vi "BuildClass.vi"(6 "ProjectPath":path, 7 "Parent":enum16{"None", "Interface", "Class"}(ring)=enum."Interface", 8 "error in (no error)":errorcluster, 9 "Application":refnum<vi>, 10 "ParentRef":refnum<vi>, 11 "Class in":refnum<class "Class.lvclass">) -> (0 "error out":errorcluster, 3 "Class out":refnum<class "Class.lvclass">)   [LabVIEW 2020, in "Mermaid.lvlib" / "Class.lvclass"]
uses:
  Class.lvclass
  Class.lvclass/Class.ctl
  _CreateClass/CreateClass.lvclass
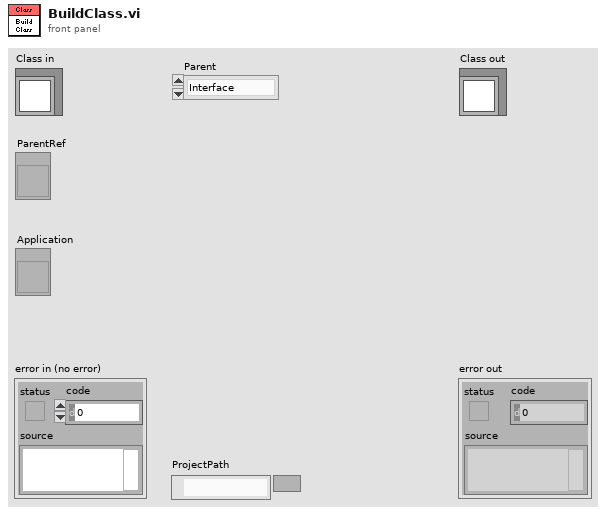
[diagram p1: front panel]
types:
  T1 = typedef "Mermaid.lvlib/ParseMermaid.lvclass/Attributes.ctl" = cluster{"Name":string, "Type":i32}[]
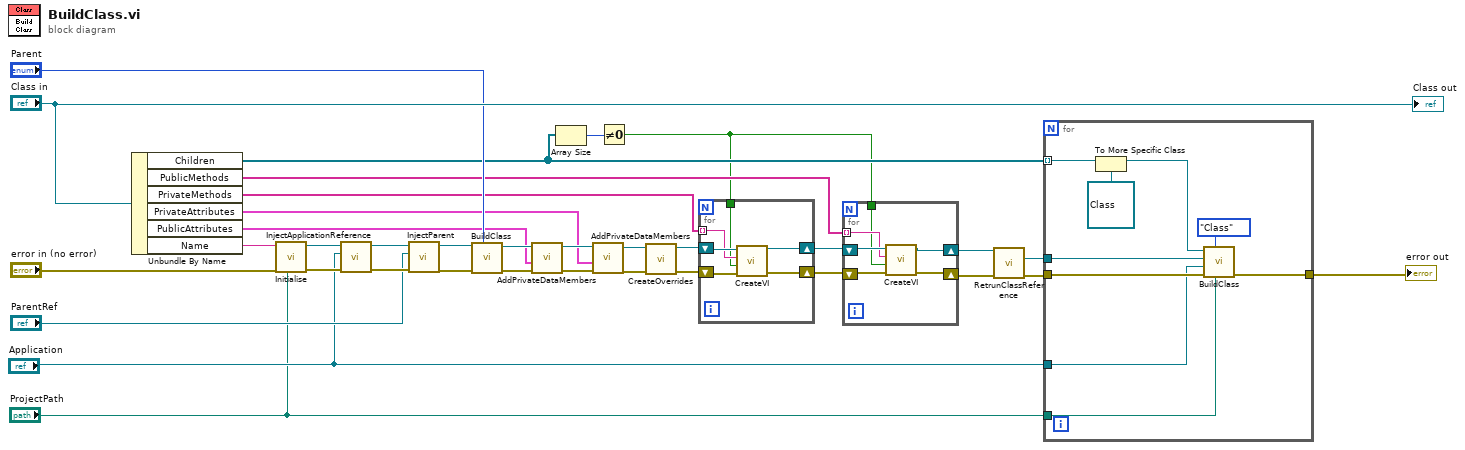
[diagram p0: block diagram]
diagram:
  n1 = Unbundle By Name("Class in") -> ("Children"=w5:refnum<class "iClass.lvclass">[], "PublicMethods"=w16:string[], "PrivateMethods"=w17:string[], "PrivateAttributes"=w20:T1, "PublicAttributes"=w21:T1, "Name"=w6:string)
  n2 = call "Initialise.vi"("ProjectPath"="ProjectPath", "error in (no error)"="error in (no error)", "Interface Name"=w6) -> ("error out"=w28:errorcluster, "Class Out"=w33:refnum<class "CreateClass.lvclass">)  [unwired: 7 in]
  n3 = call "InjectApplicationReference.vi"("error in (no error)"=w28, "Application"="Application", "CreateClass In"=w33) -> ("error out"=w29:errorcluster, "CreateClass Out"=w34:refnum<class "CreateClass.lvclass">)  [unwired: 7 in]
  n4 = call "InjectParent.vi"("error in (no error)"=w29, "Parent"="ParentRef", "CreateClass in"=w34) -> ("error out"=w30:errorcluster, "CreateClass out"=w31:refnum<class "CreateClass.lvclass">)  [unwired: 7 in]
  n5 = call "BuildClass.vi"("Parent"="Parent", "error in (no error)"=w30, "CreateClass in"=w31) -> ("error out"=w25:errorcluster, "CreateClass Out"=w24:refnum<class "CreateClass.lvclass">)  [unwired: 7 in]
  n6 = call "AddPrivateDataMembers.vi"("error in (no error)"=w25, "Class Members"=w21, "CreateClass In"=w24) -> ("error out"=w23:errorcluster, "CreateClass Ou"=w22:refnum<class "CreateClass.lvclass">)  [unwired: 7 in]
  n7 = Array Size(array=w5) -> (size(s)=w4:i32)
  n8 = call "AddPrivateDataMembers.vi"("error in (no error)"=w23, "Class Members"=w20, "CreateClass In"=w22) -> ("error out"=w14:errorcluster, "CreateClass Ou"=w15:refnum<class "CreateClass.lvclass">)  [unwired: 7 in]
  n9 = Not Equal To 0?(x=w4) -> (x != 0?=w3:bool)
  n10 = call "CreateOverrides.vi"("error in (no error)"=w14, "CreateClass in"=w15) -> ("error out"=w12:errorcluster, "CreateClass out"=w13:refnum<class "CreateClass.lvclass">)  [unwired: 8 in]
  n11 = for {
    tunnel: w17 -> [w38] mode=indexing
    shift-right: [w37] -> w19
    shift-left: w13 -> [w39]
    shift-right: [w40] -> w18
    shift-left: w12 -> [w41]
    tunnel: w3 -> [w36]
    n12 = call "CreateVI.vi"("error in (no error)"=w41, "Dynamic Dispatch (T)"=w36, "Name"=w38, "CreateClass In"=w39) -> ("error out"=w40:errorcluster, "CreateClass Out"=w37:refnum<class "CreateClass.lvclass">)  [unwired: 6 in]
  }
  n13 = for {
    tunnel: w16 -> [w43] mode=indexing
    shift-right: [w46] -> w11
    shift-left: w19 -> [w45]
    shift-right: [w47] -> w10
    shift-left: w18 -> [w44]
    tunnel: w3 -> [w42]
    n14 = call "CreateVI.vi"("error in (no error)"=w44, "Dynamic Dispatch (T)"=w42, "Name"=w43, "CreateClass In"=w45) -> ("error out"=w47:errorcluster, "CreateClass Out"=w46:refnum<class "CreateClass.lvclass">)  [unwired: 6 in]
  }
  n15 = call "RetrunClassReference.vi"("error in (no error)"=w10, "CreateClass in"=w11) -> ("error out"=w9:errorcluster, "ClassRef"=w8:refnum<vi>)  [unwired: 7 in, 1 out]
  n16 = for {
    tunnel: w9 -> [w56]
    tunnel: w8 -> [w54]
    tunnel: "Application" -> [w53]
    tunnel: w5 -> [w49] mode=indexing
    tunnel: [w52] -> w7
    tunnel: "ProjectPath" -> [w48]
    n17 = To More Specific Class(target class=refnum<class "Class.lvclass"> refnum ("Class.lvclass"), reference=w49) -> (specific class reference=w51:refnum<class "Class.lvclass">)  [unwired: 1 in, 1 out]
    n18 = call-dynamic "BuildClass.vi"("ProjectPath"=w48, "Parent"=enum16{"None", "Interface", "Class"}."Class", "error in (no error)"=w56, "Application"=w53, "ParentRef"=w54, "Class in"=w51) -> ("error out"=w52:errorcluster)  [unwired: 4 in, 1 out]
  }
  "error out" <- w7
  "Class out" <- "Class in"
